vi "logUser.vi"(8 "error in (no error)":errorcluster, 9 "pass":string, 10 "user":string, 11 "Usuarios in":refnum<class "Usuarios.lvclass">) -> (0 "error out":errorcluster, 3 "Usuarios out":refnum<class "Usuarios.lvclass">)   [LabVIEW 2019, in "Usuarios.lvclass"]
uses:
  Usuarios.lvclass
panel:
  in  "OK":bool
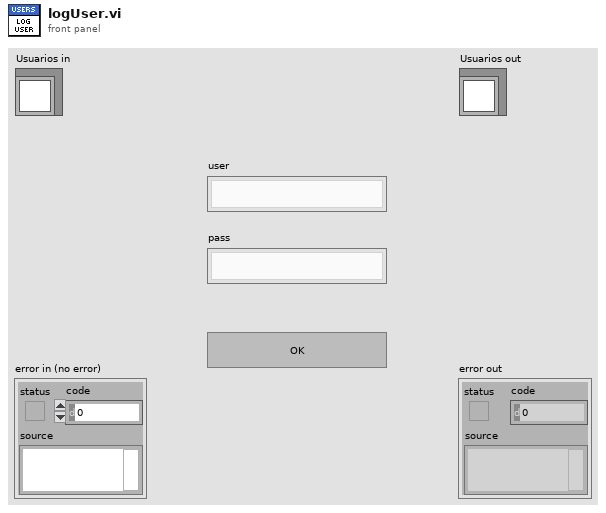
[diagram p1: front panel]
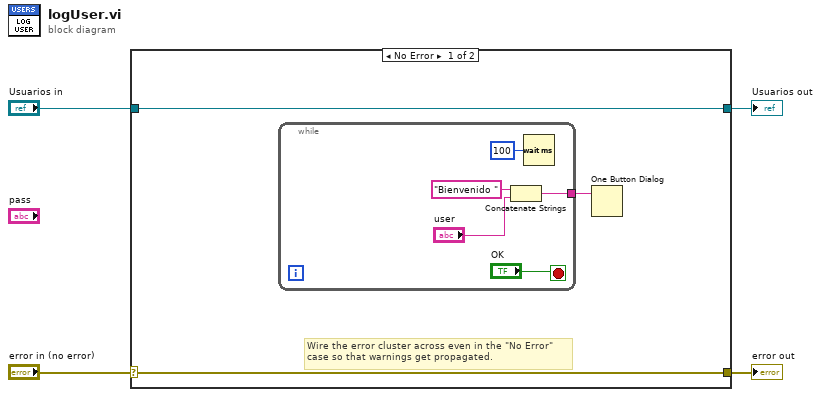
[diagram p0: block diagram]
diagram:
  n1 = case shown="No Error" "error in (no error)" {
    selector: "error in (no error)" -> [w6 w14]
    tunnel: [w6 w14] -> w3
    tunnel: [w7 w13] -> w1
    tunnel: "Usuarios in" -> [w7 w13]
    frame No Error {
      # "Wire the error cluster across even in the \"No Error\"\ncase so that warnings get propagated."
      n2 = while {
        tunnel: [w9] -> w5
        stop <- "OK" stop-if-true
        n3 = Concatenate Strings("Bienvenido " ("string"), "user") -> (w9:string)
        n4 = Wait (ms)(milliseconds to wait=u32 100) -> ()  [unwired: 1 out]
      }
      n5 = One Button Dialog(message=w5) -> ()  [unwired: 1 in, 1 out]
    }
    frame Error {
    }
  }
  "error out" <- w3
  "Usuarios out" <- w1
